vi "Status.vi"(8 "error in":errorcluster, 10 "State":T1(ring), 11 "Operation":enum16{"Initialize", "Set Status", "Shutdown"}(ring)=enum."Set Status") -> (0 "error out":errorcluster)   [LabVIEW 2026, in "NIVS_CDEW_MetaDataObj.lvclass"]
uses:
  NIVS_CDEW_MetaDataObj.lvclass
  Status Dialog.vi
  NIVS_CDEW_MetaDataObj.lvclass/NIVS_CDEW_MetaDataObj.ctl
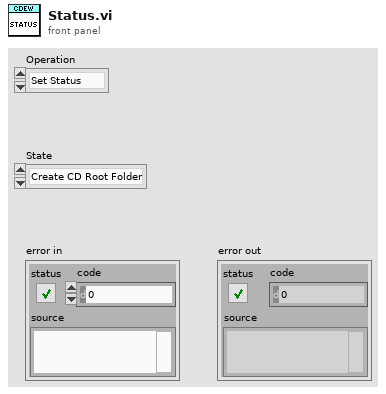
[diagram p1: front panel]
types:
  T1 = enum16{"Create CD Root Folder", "Copy Compiled Settings", "Generate Custom Device DLL from XML", "Calculate Page Properties", "Create Configuration Project", "Create Engine Project", "Create Custom Device Engine Project", "Create System Explorer Project", "Create Test Hooks Project", "Relink and Clean Up VIs", "Build PPLs", "Copy Custom Device DLL to Public Documents", "Open Projects", "Shutdown"}
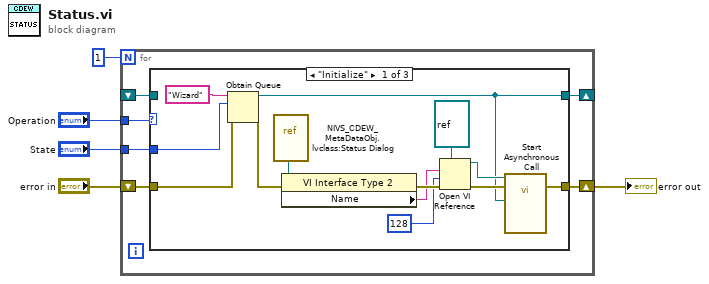
[diagram p0: block diagram]
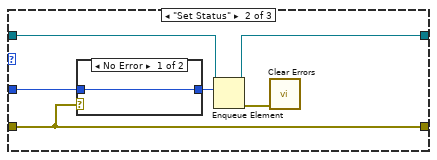
[diagram p2: hidden frame]
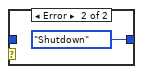
[diagram p3: hidden frame]
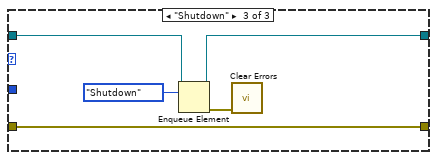
[diagram p4: hidden frame]
diagram:
  n1 = for {
    N: 1 -> [_]
    tunnel: "Operation" -> [w9]
    shift-right: [w8] -> _
    shift-left: _ -> [w7]
    shift-right: [w10] -> w4
    shift-left: "error in" -> [w11]
    tunnel: "State" -> [w6]
    n2 = case shown="\"Initialize\"" w9 {
      tunnel: [w12 w26 w34] -> w8
      tunnel: w7 -> [_ w28 w35]
      tunnel: w11 -> [w24 w30 w37]
      tunnel: [w22 w30 w37] -> w10
      tunnel: w6 -> [w18 w25 _]
      frame "Initialize" {
        n3 = Obtain Queue(name (unnamed)="Wizard", element data type=w18, error in (no error)=w24) -> (queue out=w12:refnum<queue>, error out=w20:errorcluster)  [unwired: 2 in, 1 out]
        n4 = vi-ref "NIVS_CDEW_MetaDataObj.lvclass:Status Dialog.vi"() -> (w16:refnum<vi>)
        n5 = property class="VI Interface Type 2"(reference=w16, error in=w20) -> (error out=w21:errorcluster, "Name"=w15:string)  [unwired: 1 out]
        n6 = Open VI Reference(type specifier VI Refnum (for type only)=refnum<vi> refnum, vi path=w15, options=128, error in (no error)=w21) -> (vi reference=w14:refnum<vi>, error out=w23:errorcluster)  [unwired: 2 in]
        n7 = call-by-ref "Start Asynchronous Call"(reference=w14, error in=w23, "queue in"=w12) -> (error out=w22:errorcluster)  [unwired: 11 in, 1 out]
      }
      frame "Set Status" {
        n8 = case shown="No Error" w30 {
          tunnel: [w31 T1."Shutdown" ("element")] -> w27
          tunnel: w25 -> [w31 _]
          frame No Error {
          }
          frame Error {
          }
        }
        n9 = Enqueue Element(queue=w28, element=w27) -> (queue out=w26:refnum<queue>, error out=w29:errorcluster)  [unwired: 2 in, 1 out]
        n10 = call <vilib>:"Clear Errors.vi"("error in (no error)"=w29) -> ()  [unwired: 5 in, 2 out]
      }
      frame "Shutdown" {
        n11 = Enqueue Element(queue=w35, element=T1."Shutdown") -> (queue out=w34:refnum<queue>, error out=w36:errorcluster)  [unwired: 2 in, 1 out]
        n12 = call <vilib>:"Clear Errors.vi"("error in (no error)"=w36) -> ()  [unwired: 5 in, 2 out]
      }
    }
  }
  "error out" <- w4
